vi "test_SetItemInfoDependencies_SampleProjectWithExternalDep.vi"() -> (3 "Pass?":bool)   [LabVIEW 2019, in "Tests.SolutionBuilder.lvlib"]
uses:
  Tests.SolutionBuilder.lvlib
  SolutionBuilder/SolutionBuilder.lvclass
  SolutionBuilder/ProjectItem/ProjectItem.lvclass
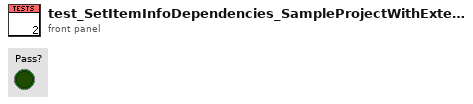
[diagram p1: front panel]
types:
  T1 = cluster{"Relative Path from 1 to 2":path, string[]}
  T2 = typedef "SolutionBuilder.lvlib/SolutionBuilder.lvclass/ProjectItemMap.ctl" = map{path, refnum<class "ProjectItem.lvclass">[]}
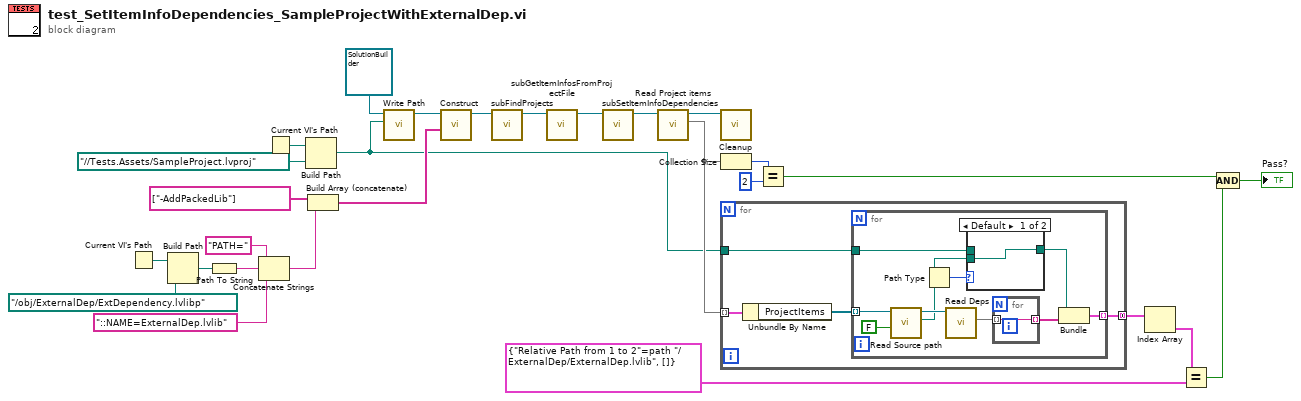
[diagram p0: block diagram]
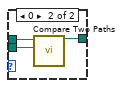
[diagram p2: hidden frame]
diagram:
  n1 = Current VI's Path() -> (path=w11:path)
  n2 = Build Path(base path=w11, name or relative path=path "../obj/ExternalDep/ExtDependency.lvlibp" ("Path")) -> (appended path=w13:path)
  n3 = Path To String(path=w13) -> (string=w7:string)
  n4 = Concatenate Strings("PATH=", w7, "::NAME=ExternalDep.lvlib") -> (w8:string)
  n5 = Current VI's Path() -> (path=w26:path)
  n6 = Build Path(base path=w26, name or relative path=path "../../Tests.Assets/SampleProject.lvproj" ("Path")) -> (appended path=w9:path)
  n7 = Build Array (concatenate)(string[] ["-AddPackedLib"] ("App.Args"), w8) -> (w12:string[])
  n8 = call "Write Path.vi"("Path"=w9, "SolutionBuilder in"=refnum<class "SolutionBuilder.lvclass"> refnum) -> ("SolutionBuilder out"=w18:refnum<class "SolutionBuilder.lvclass">)  [unwired: 9 in]
  n9 = call "Construct.vi"("App.Args"=w12, "SolutionBuilder in"=w18) -> ("SolutionBuilder out"=w17:refnum<class "SolutionBuilder.lvclass">)  [unwired: 8 in, 1 out]
  n10 = call "subFindProjects.vi"("SolutionBuilder in"=w17) -> ("SolutionBuilder out"=w27:refnum<class "SolutionBuilder.lvclass">)  [unwired: 9 in, 1 out]
  n11 = call "subGetItemInfosFromProjectFile.vi"("SolutionBuilder in"=w27) -> ("SolutionBuilder out"=w20:refnum<class "SolutionBuilder.lvclass">)  [unwired: 9 in, 1 out]
  n12 = call "subSetItemInfoDependencies.vi"("SolutionBuilder in"=w20) -> ("SolutionBuilder out"=w19:refnum<class "SolutionBuilder.lvclass">)  [unwired: 9 in, 1 out]
  n13 = call "Read Project items.vi"("SolutionBuilder in"=w19) -> ("Project items"=w22:T2, "SolutionBuilder out"=w16:refnum<class "SolutionBuilder.lvclass">)  [unwired: 9 in]
  n14 = call "Cleanup.vi"("SolutionBuilder in"=w16) -> ()  [unwired: 9 in, 2 out]
  n15 = Collection Size(1:w22) -> (0:w24:i32)
  n16 = for {
    tunnel: w22 -> [w32] mode=indexing
    tunnel: [w30] -> w4 mode=concatenating
    tunnel: w9 -> [w29]
    n17 = Unbundle By Name(w32) -> ("ProjectItems"=w31:refnum<class "ProjectItem.lvclass">[])
    n18 = for {
      tunnel: w31 -> [w39] mode=indexing
      tunnel: [w40] -> w30 mode=indexing
      tunnel: w29 -> [w33]
      n19 = call "Read Source path.vi"("Force abs path? (T)"=FALSE, "ProjectItem in"=w39) -> ("Source path"=w35:path, "ProjectItem out"=w38:refnum<class "ProjectItem.lvclass">)  [unwired: 8 in]
      n20 = Path Type(1:w35) -> (0:w36:i16)
      n21 = call "Read Deps.vi"("ProjectItem in"=w38) -> ("Deps"=w42:set{string})  [unwired: 9 in, 1 out]
      n22 = case shown="Default" w36 {
        tunnel: w35 -> [w43 w44]
        tunnel: [w43 w46] -> w34
        tunnel: w33 -> [_ w45]
        frame Default {
        }
        frame 0 {
          n23 = call <vilib>:"Compare Two Paths.vi"("Path 2"=w44, "Path 1"=w45) -> ("Relative Path from 1 to 2"=w46:path)  [unwired: 6 in, 3 out]
        }
      }
      n24 = for {
        tunnel: w42 -> [w47] mode=indexing
        tunnel: [w47] -> w41 mode=indexing
      }
      n25 = Bundle("Relative Path from 1 to 2"=w34, w41) -> (w40:T1)  [unwired: 1 in]
    }
  }
  n26 = Equal?(x=w24, y=2) -> (x = y?=w21:bool)
  n27 = Index Array(array=w4) -> (element=w3:T1)  [unwired: 1 in]
  n28 = Equal?(x=w3, y=T1 {"Relative Path from 1 to 2"=path "../ExternalDep/ExternalDep.lvlib", []}) -> (x = y?=w15:bool)
  n29 = Compound Arithmetic op=AND(w21, w15) -> (→"Pass?":bool)
